vi "send.vi"(0 "HGF_Queue":refnum<class "HGF_Queue.lvclass">, 2 "Object":refnum<class>, 3 "timeout in ms (-1)":i32, 5 "error in (no error)":errorcluster, 9 "mode (Queue)":bool) -> (14 "HGF_Queue":refnum<class "HGF_Queue.lvclass">, 17 "timed out?":bool, 19 "error out":errorcluster)   [LabVIEW 2014, in "HGF_BaseClasses.lvlib" / "HGF_Queue.lvclass"]
doc: "Send an object.\n\nHint: This is a dynamic dispatch VI to be implemented by the child class."
uses:
  HGF_Queue.lvclass
  HGF_Auxiliary/HGF_Auxiliary.lvlib
  HGF_Auxiliary/Severity.ctl
  HGF_Auxiliary/ErrorCode.ctl
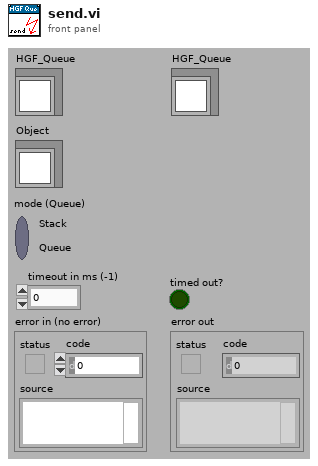
[diagram p1: front panel]
types:
  T1 = typedef "HGF_Auxiliary.lvlib/ErrorCode.ctl" = enum32{"No error", "Function not supported.", "This VI is for friends only.", "Reference object aready exisits.", "Parameter out of range.", "Not a rendezvous.", "Invalid notifier reference.", "Invalid queue reference.", "Self-Test not supported.", "Reset not supported.", "IDN query not supported.", "Error query not supported.", "Incorrect addressee.", "Object already exists.", "No class name specified", "Driver not supported", "Attribute is not writable"}
  T2 = typedef "HGF_Auxiliary.lvlib/Severity.ctl" = enum16{"Info", "Warning", "Fault", "Error", "Fatal"}
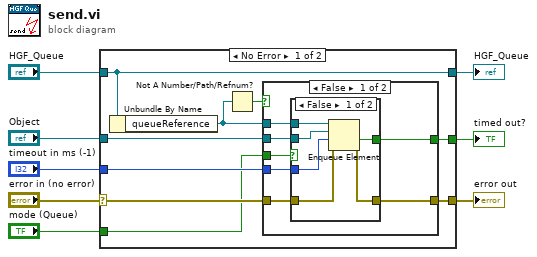
[diagram p0: block diagram]
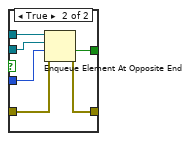
[diagram p2: hidden frame]
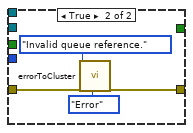
[diagram p3: hidden frame]
diagram:
  n1 = case shown="No Error" "error in (no error)" {
    selector: "error in (no error)" -> [w13 w41]
    tunnel: "HGF_Queue" -> [w12 w42]
    tunnel: "Object" -> [w17 _]
    tunnel: "timeout in ms (-1)" -> [w16 _]
    tunnel: [w15 w41] -> w5
    tunnel: [w14 _] -> w4
    tunnel: [w12 w42] -> w2
    tunnel: "mode (Queue)" -> [w11 _]
    frame No Error {
      n2 = Unbundle By Name(w12) -> ("queueReference"=w9:refnum<queue>)
      n3 = Not A Number/Path/Refnum?(number/path/refnum=w9) -> (NaN/Path/Refnum?=w10:bool)
      n4 = case shown="False" w10 {
        tunnel: w9 -> [w24 _]
        tunnel: w17 -> [w23 _]
        tunnel: w16 -> [w22 _]
        tunnel: [w21 w39] -> w15
        tunnel: [w20 _] -> w14
        tunnel: w13 -> [w19 w40]
        tunnel: w11 -> [w18 _]
        frame False {
          n5 = case shown="False" w18 {
            tunnel: w24 -> [w30 w36]
            tunnel: w23 -> [w29 w35]
            tunnel: w22 -> [w28 w34]
            tunnel: [w27 w32] -> w21
            tunnel: [w26 w33] -> w20
            tunnel: w19 -> [w25 w31]
            frame False {
              n6 = Enqueue Element(queue=w30, element=w29, timeout in ms (-1)=w28, error in (no error)=w25) -> (timed out?=w26:bool, error out=w27:errorcluster)  [unwired: 1 out]
            }
            frame True {
              n7 = Enqueue Element At Opposite End(queue=w36, element=w35, timeout in ms (-1)=w34, error in (no error)=w31) -> (timed out?=w33:bool, error out=w32:errorcluster)  [unwired: 1 out]
            }
          }
        }
        frame True {
          n8 = call "errorToCluster.vi"("error code"=ErrorCode."Invalid queue reference." ("HGF_Error"), "error in (no error)"=w40, "severity (Error)"=Severity."Error") -> ("error out"=w39:errorcluster)  [unwired: 2 in, 14 out]
        }
      }
    }
    frame Error {
    }
  }
  "error out" <- w5
  "HGF_Queue" <- w2
  "timed out?" <- w4
